vi "get Plot String.vi"(8 "error in (no error)":errorcluster) -> (0 "error out":errorcluster, 3 "function return":string)   [LabVIEW 2019, in "libOutputReader.lvlib"]
doc: "const char* getPlotString();"
uses:
  libOutputReader.lvlib
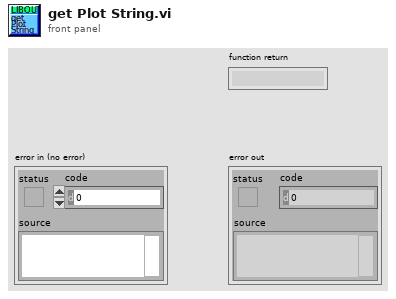
[diagram p1: front panel]
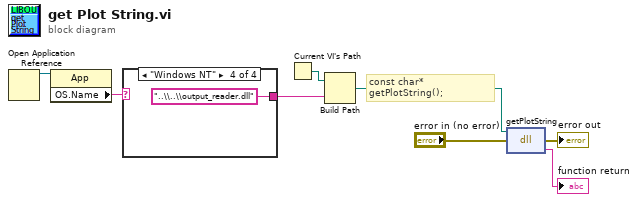
[diagram p0: block diagram]
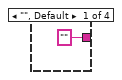
[diagram p2: hidden frame]
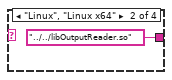
[diagram p3: hidden frame]
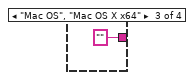
[diagram p4: hidden frame]
diagram:
  # "const char* getPlotString();"
  n1 = Open Application Reference() -> (3:w4:refnum<vi>)  [unwired: 4 in, 1 out]
  n2 = property class="App"(reference=w4) -> ("OS.Name"=w3:string)  [unwired: 1 in, 2 out]
  n3 = case shown="\"Windows NT\"" w3 {
    tunnel: ["" ("return type") "../../libOutputReader.so" ("name or relative path") "" ("return type") "..\\..\\output_reader.dll" ("name or relative path")] -> w2
    frame "", Default {
    }
    frame "Linux", "Linux x64" {
    }
    frame "Mac OS", "Mac OS X x64" {
    }
    frame "Windows NT" {
    }
  }
  n4 = Current VI's Path() -> (path=w5:path)
  n5 = Build Path(base path=w5, name or relative path=w2) -> (appended path=w1:path)
  n6 = dll-call lib="home/paul/Schreibtisch/Biogas_plant_setup/LabView/lib/libOutputReader/libOutputReader.*" fn="getPlotString"(path in=w1, error in="error in (no error)") -> (error out=→"error out":errorcluster, "return type"=→"function return":string)  [unwired: 1 in, 1 out]
